vi "Read Long.vi"(11 "GDSII.DataType in":refnum<class "GDSII.DataType.lvclass">) -> (2 "Long":i32[](array[numeric]), 3 "GDSII.DataType out":refnum<class "GDSII.DataType.lvclass">)   [LabVIEW 2019, in "GDSII.DataType.lvclass"]
uses:
  GDSII.DataType.lvclass
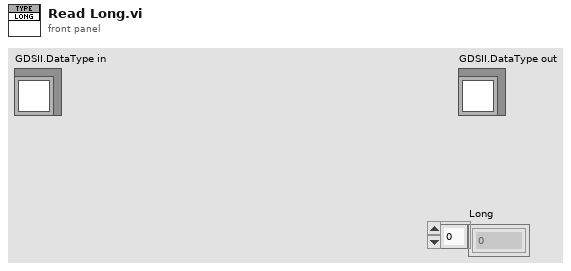
[diagram p1: front panel]
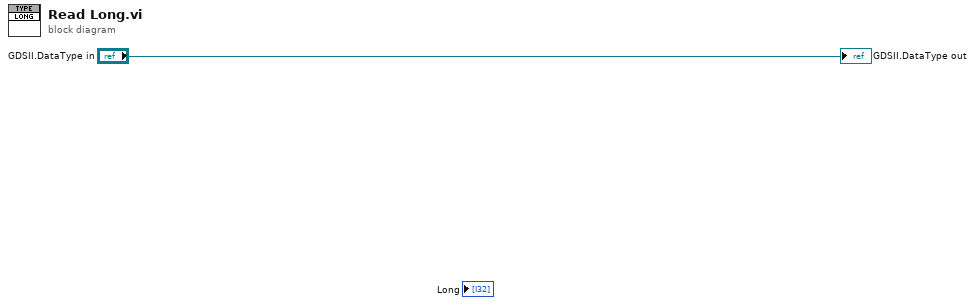
[diagram p0: block diagram]
diagram:
  "GDSII.DataType out" <- "GDSII.DataType in"
